vi "Find Object Item Locations by Names.vi"(5 "Insertion point if not found":bool, 6 "Only return first found":bool, 7 "Item Names <JSON>":string[](array[string]), 8 "error in (no error)":errorcluster, 10 "Object Offset":i32, 11 "JSON":string) -> (0 "error out":errorcluster, 1 "Items":T1[](array[typedef]))   [LabVIEW 2017, in "JSONtext.lvlib"]
uses:
  JSONtext.lvlib
  Parsing/Found Items.ctl
  Parsing/Parsing State.ctl
  Parsing/Advance past String.vi
  Parsing/Advance past Number.vi
  Parsing/Advance past Object.vi
  Parsing/Advance past Array.vi
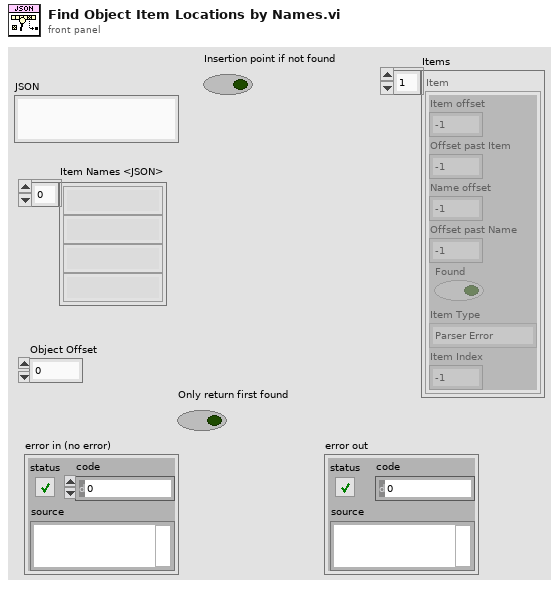
[diagram p1: front panel]
types:
  T1 = typedef "JSONtext.lvlib/Found Items.ctl" = cluster{"Item offset":i32, "Offset past Item":i32, "Name offset":i32, "Offset past Name":i32, "Found":bool, "Item Type":T2, "Item Index":i32}
  T2 = typedef "JSONtext.lvlib/Parsing State.ctl" = enum16{"Parser Error", "Object", "Array", "String", "Number/Other", "Leading Whitespace", "Object end", "Array end", "Value end"}
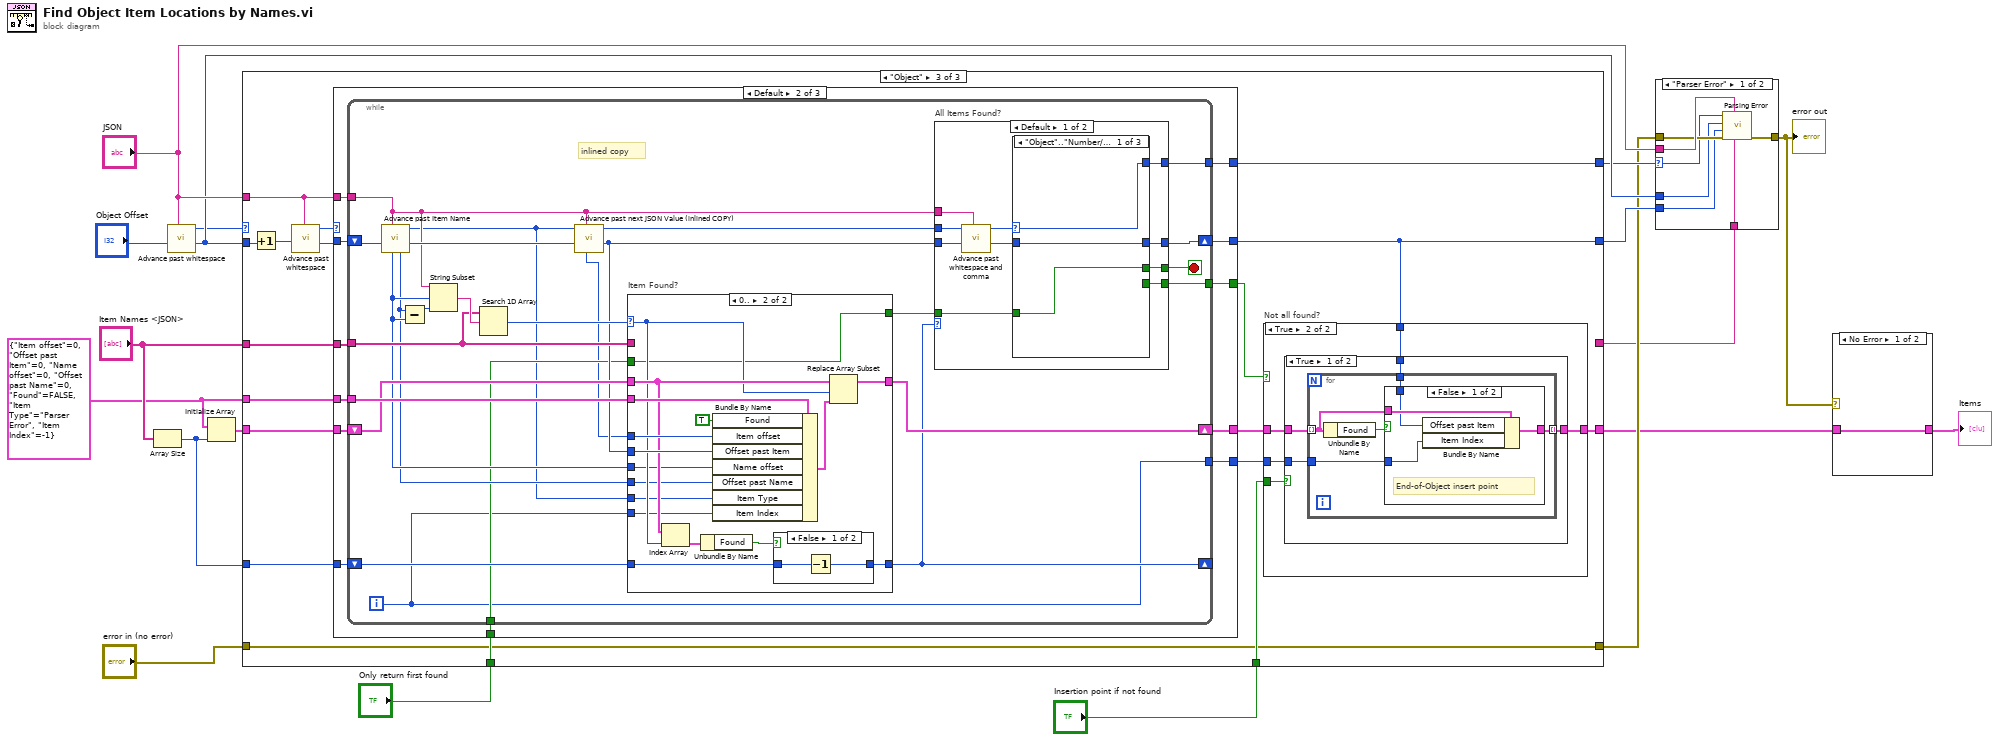
[diagram p0: block diagram]
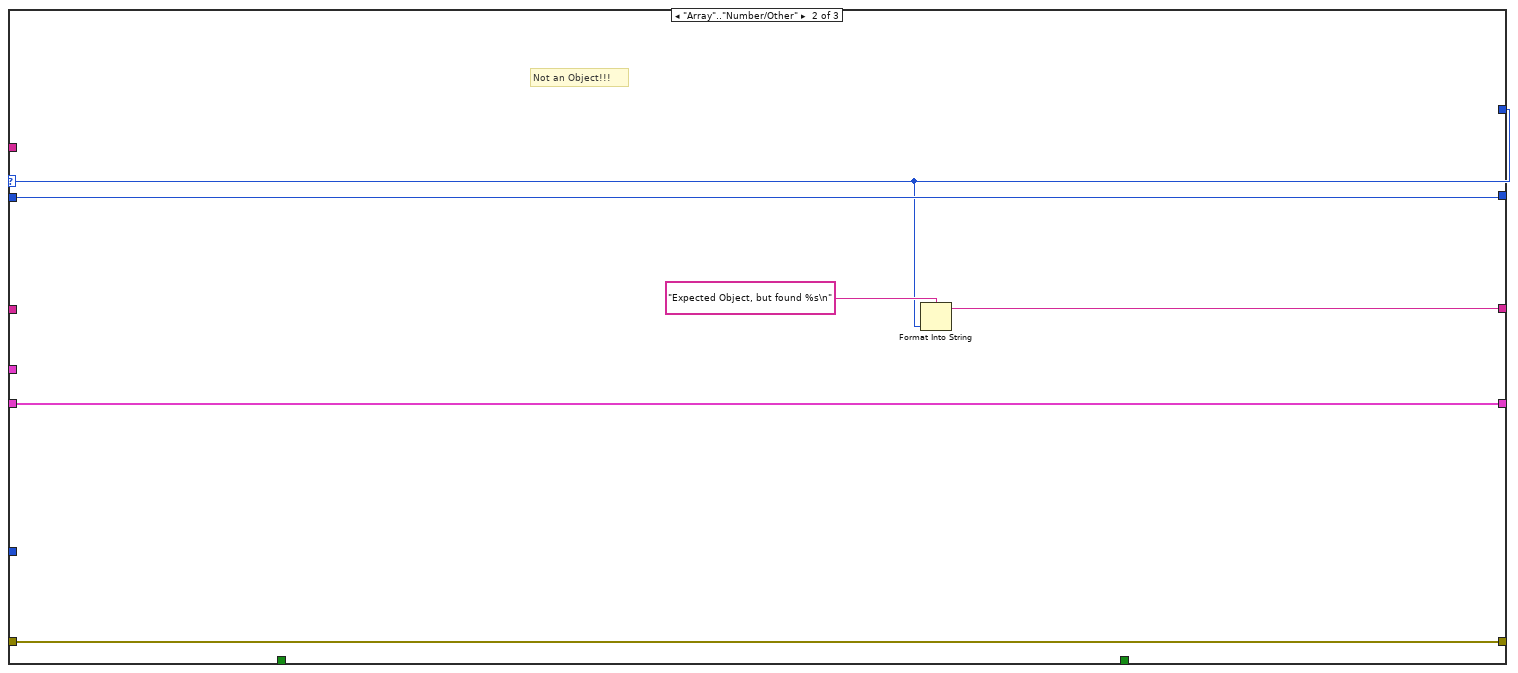
[diagram p3: hidden frame]
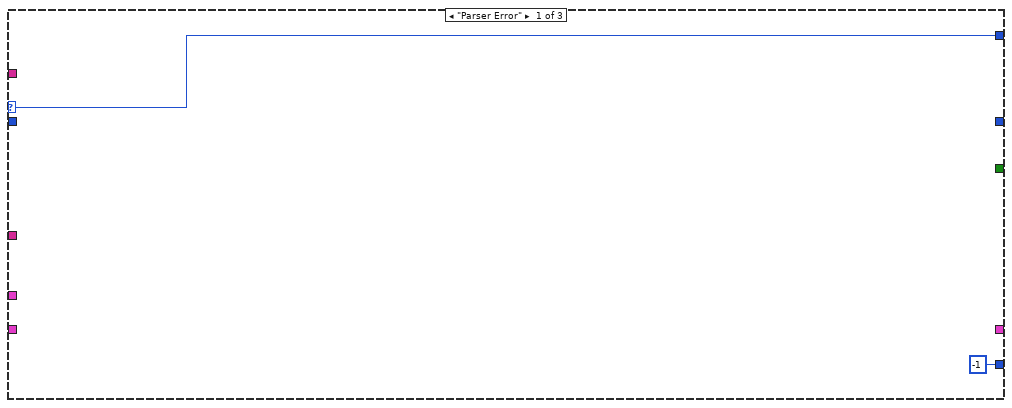
[diagram p4: hidden frame]
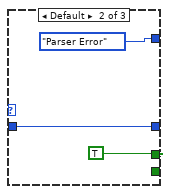
[diagram p7: hidden frame]
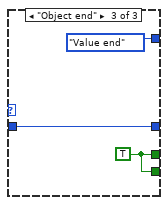
[diagram p8: hidden frame]
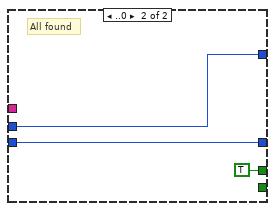
[diagram p9: hidden frame]
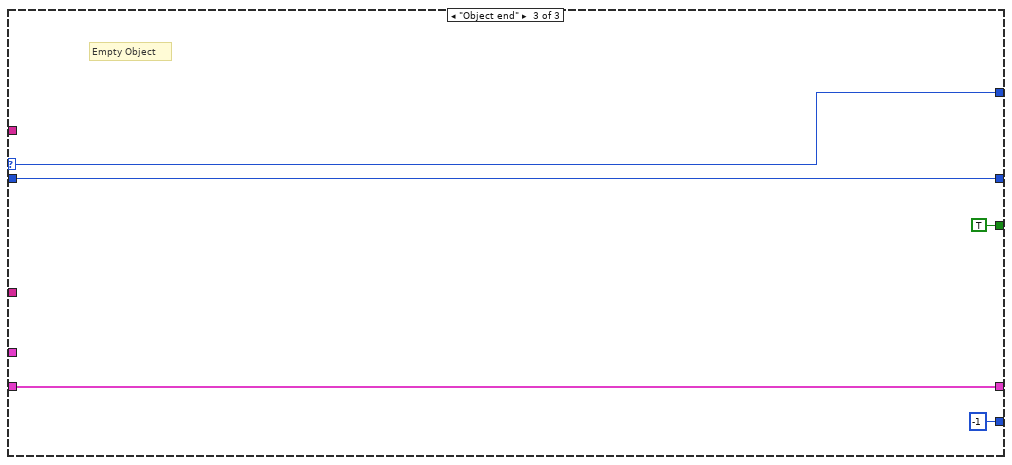
[diagram p10: hidden frame]
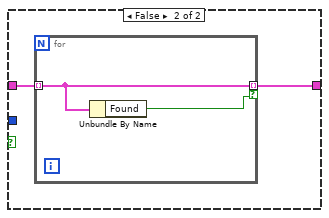
[diagram p13: hidden frame]
diagram:
  w15 = T1 {"Item offset"=0, "Offset past Item"=0, "Name offset"=0, "Offset past Name"=0, "Found"=FALSE, "Item Type"=enum."Parser Error", "Item Index"=-1}
  n1 = Array Size(array="Item Names <JSON>") -> (size(s)=w14:i32)
  n2 = call "Advance past whitespace.vi"("JSON"="JSON", "Offset"="Object Offset") -> ("Offset of first non-whitespace"=w11:i32, "Parser State"=w10:T2)  [unwired: 8 in]
  n3 = Initialize Array(w15, w14) -> (w16:T1[])
  n4 = case shown="\"Object\"" w10 {
    selector: w10 -> [w19 w24 _]
    tunnel: "Item Names <JSON>" -> [_ _ w46]
    tunnel: w16 -> [w22 w28 w45]
    tunnel: w15 -> [_ _ w44]
    tunnel: w14 -> [_ _ w43]
    tunnel: [w22 w28 w40] -> w2
    tunnel: "JSON" -> [_ _ w32]
    tunnel: [w20 w26 w39] -> w12
    tunnel: w11 -> [w20 w26 w38]
    tunnel: [w19 w24 w37] -> w9
    tunnel: "Only return first found" -> [_ _ w36]
    tunnel: "Insertion point if not found" -> [_ _ w35]
    tunnel: "error in (no error)" -> [w21 w27 w34]
    tunnel: [w21 w27 w34] -> w5
    tunnel: [_ w23 _] -> w1
    frame "Parser Error", Default {
      # "Not an Object!!!"
    }
    frame "Array".."Number/Other" {
      # "Not an Object!!!"
      n5 = Format Into String(format string="Expected Object, but found %s\n", w24) -> (resulting string=w23:string)  [unwired: 2 in, 1 out]
    }
    frame "Object" {
      n6 = Increment(x=w38) -> (x+1=w33:i32)
      n7 = call "Advance past whitespace.vi"("JSON"=w32, "Offset"=w33) -> ("Offset of first non-whitespace"=w31:i32, "Parser State"=w30:T2)  [unwired: 8 in]
      n8 = case shown="Default" w30 {
        selector: w30 -> [w48 _ w133]
        tunnel: w31 -> [_ w60 w132]
        tunnel: w46 -> [_ w59 _]
        tunnel: w45 -> [_ w58 w131]
        tunnel: w44 -> [_ w57 _]
        tunnel: w43 -> [_ w56 _]
        tunnel: [_ w55 w131] -> w42
        tunnel: [_ w54 TRUE] -> w41
        tunnel: w32 -> [_ w53 _]
        tunnel: [_ w52 w132] -> w39
        tunnel: [w48 w51 w133] -> w37
        tunnel: w36 -> [_ w50 _]
        tunnel: [-1 w49 -1] -> w29
        frame "Parser Error" {
        }
        frame Default {
          n9 = while {
            shift-right: [w85] -> w52
            shift-left: w60 -> [w82]
            tunnel: w53 -> [w79]
            tunnel: [w83] -> w51
            tunnel: w59 -> [w74]
            tunnel: w57 -> [w76]
            shift-right: [w72] -> w55
            shift-left: w58 -> [w73]
            shift-right: [w70] -> _
            shift-left: w56 -> [w71]
            tunnel: [w68] -> w54
            tunnel: w50 -> [w65]
            tunnel: [w61] -> w49
            i -> [w61]
            stop <- w84 stop-if-true
            # "inlined copy"
            n10 = call "Advance past Item Name.vi"("JSON"=w79, "Offset"=w82) -> ("Offset past colon"=w80:i32, "State"=w62:T2, "Offset past Name"=w66:i32, "Name start out"=w67:i32)  [unwired: 6 in]
            n11 = Subtract(x=w66, y=w67) -> (x-y=w78:i32)
            n12 = String Subset(string=w79, offset (0)=w67, length (rest)=w78) -> (substring=w77:string)
            n13 = Search 1D Array(1D array=w74, element=w77) -> (index of element=w75:i32)  [unwired: 1 in]
            n14 = call "Advance past next JSON Value (inlined COPY).vi"("JSON"=w79, "Offset"=w80, "State"=w62) -> ("Offset"=w69:i32, "State"=w81:T2, "Value start"=w63:i32)  [unwired: 4 in, 2 out]
            n15 = case "Item Found?" shown="0.." w75 {
              selector: w75 -> [_ w98]
              tunnel: w76 -> [_ w104]
              tunnel: w63 -> [_ w102]
              tunnel: w69 -> [_ w101]
              tunnel: w74 -> [_ _]
              tunnel: w73 -> [w87 w99]
              tunnel: [w87 w97] -> w72
              tunnel: w71 -> [w86 w94]
              tunnel: [w86 w93] -> w70
              tunnel: w67 -> [_ w92]
              tunnel: w66 -> [_ w91]
              tunnel: w65 -> [_ w90]
              tunnel: [_ w90] -> w64
              tunnel: w62 -> [_ w89]
              tunnel: w61 -> [_ w88]
              frame Default {
              }
              frame 0.. {
                n16 = Index Array(array=w99, index=w98) -> (element=w96:T1)
                n17 = Unbundle By Name(w96) -> ("Found"=w95:bool)
                n18 = Bundle By Name(cluster=w104, "Found"=TRUE, "Item offset"=w102, "Offset past Item"=w101, "Name offset"=w92, "Offset past Name"=w91, "Item Type"=w89, "Item Index"=w88) -> (w100:T1)
                n19 = case shown="False" w95 {
                  tunnel: w94 -> [w106 w107]
                  tunnel: [w105 w107] -> w93
                  frame False {
                    n20 = Decrement(x=w106) -> (x-1=w105:i32)
                  }
                  frame True {
                  }
                }
                n21 = Replace Array Subset(array=w99, new element=w100, index=w98) -> (w97:T1[])
              }
            }
            n22 = case "All Items Found?" shown="Default" w70 {
              tunnel: [w116 w128] -> w85
              tunnel: [w115 TRUE] -> w84
              tunnel: [w114 w129] -> w83
              tunnel: w81 -> [w109 w129]
              tunnel: w69 -> [w112 w128]
              tunnel: w79 -> [w113 _]
              tunnel: [w110 _] -> w68
              tunnel: w64 -> [w108 _]
              frame Default {
                n23 = call "Advance past whitespace and comma.vi"("JSON"=w113, "Offset"=w112, "State in"=w109) -> ("Offset past match"=w111:i32, "State"=w117:T2)  [unwired: 7 in]
                n24 = case shown="\"Object\"..\"Number/Other\"" w117 {
                  selector: w117 -> [w118 _ _]
                  tunnel: [w119 TRUE w125] -> w115
                  tunnel: [w118 Parsing_State."Parser Error" Parsing_State."Value end"] -> w114
                  tunnel: w111 -> [w120 w121 w124]
                  tunnel: [w120 w121 w124] -> w116
                  tunnel: [_ _ w125] -> w110
                  tunnel: w108 -> [w119 _ _]
                  frame "Object".."Number/Other" {
                  }
                  frame Default {
                  }
                  frame "Object end" {
                    w125 = TRUE
                  }
                }
              }
              frame ..0 {
                # "All found"
              }
            }
          }
        }
        frame "Object end" {
          # "Empty Object"
        }
      }
      n25 = case "Not all found?" shown="True" w41 {
        tunnel: w42 -> [w135 w140]
        tunnel: [w135 w139] -> w40
        tunnel: w39 -> [_ w138]
        tunnel: w35 -> [_ w137]
        tunnel: w29 -> [_ w136]
        frame False {
        }
        frame True {
          n26 = case shown="True" w137 {
            tunnel: w140 -> [w145 w157]
            tunnel: [w144 w156] -> w139
            tunnel: w138 -> [w143 _]
            tunnel: w136 -> [w142 _]
            frame True {
              n27 = Increment(x=w142) -> (x+1=w141:i32)
              n28 = for {
                tunnel: w145 -> [w148] mode=indexing
                tunnel: [w149] -> w144 mode=indexing
                tunnel: w143 -> [w147]
                tunnel: w141 -> [w146]
                n29 = Unbundle By Name(w148) -> ("Found"=w150:bool)
                n30 = case shown="False" w150 {
                  tunnel: [w153 w155] -> w149
                  tunnel: w148 -> [w154 w155]
                  tunnel: w147 -> [w152 _]
                  tunnel: w146 -> [w151 _]
                  frame False {
                    # "End-of-Object insert point"
                    n31 = Bundle By Name(cluster=w154, "Offset past Item"=w152, "Item Index"=w151) -> (w153:T1)
                  }
                  frame True {
                  }
                }
              }
            }
            frame False {
              n32 = for {
                tunnel: w157 -> [w159] mode=indexing
                tunnel: [w159] -> w156 mode=indexing if=w158
                n33 = Unbundle By Name(w159) -> ("Found"=w158:bool)
              }
            }
          }
        }
      }
    }
  }
  n34 = case shown="\"Parser Error\"" w9 {
    selector: w9 -> [w161 _]
    tunnel: "JSON" -> [w166 _]
    tunnel: w5 -> [w165 w167]
    tunnel: [w164 w167] -> w4
    tunnel: w11 -> [w163 _]
    tunnel: w12 -> [w162 _]
    tunnel: w1 -> [w160 _]
    frame "Parser Error" {
      n35 = call "Parsing Error.vi"("initial string"=w160, "JSON"=w166, "error in (no error)"=w165, "Offset past match"=w162, "Value start"=w163, "State"=w161) -> ("error out"=w164:errorcluster)  [unwired: 5 in]
    }
    frame Default {
    }
  }
  "error out" <- w4
  n36 = case shown="No Error" w4 {
    tunnel: [w168 _] -> w3
    tunnel: w2 -> [w168 _]
    frame No Error {
    }
    frame Error {
    }
  }
  "Items" <- w3
